vi "address_plus_laserNumber_U32_to_hex.vi"(8 "adress offset":u32=300, 9 "y 3":u32=300) -> (2 "string 5":string)   [LabVIEW 2021]
panel:
  in  "string 6":string
  out "x-y*floor(x/y) 9":u32=2
  out "appended array 3":u32[](array[numeric])
  out "x-y*floor(x/y) 8":u32=2
  out "x-y*floor(x/y) 6":u32=2
  out "x-y*floor(x/y) 7":u32=12
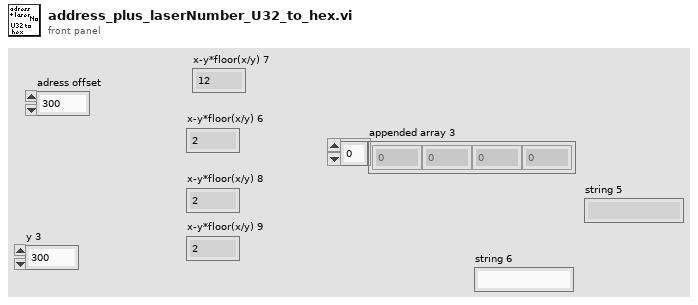
[diagram p1: front panel]
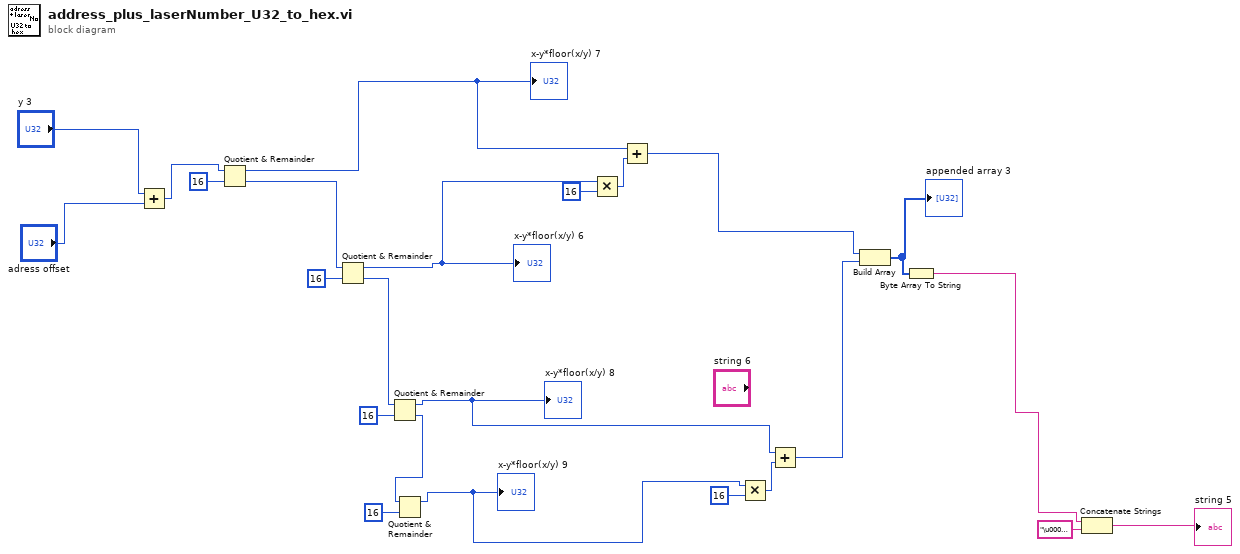
[diagram p0: block diagram]
diagram:
  n1 = Add(x="y 3", y="adress offset") -> (x+y=w6:u32)
  n2 = Quotient & Remainder(x=w6, y=u32 16) -> (x-y*floor(x/y)=w14:u32, floor(x/y)=w24:u32)
  "x-y*floor(x/y) 7" <- w14
  n3 = Quotient & Remainder(x=w24, y=u32 16) -> (x-y*floor(x/y)=w17:u32, floor(x/y)=w20:u32)
  "x-y*floor(x/y) 6" <- w17
  n4 = Quotient & Remainder(x=w20, y=u32 16) -> (x-y*floor(x/y)=w11:u32, floor(x/y)=w18:u32)
  "x-y*floor(x/y) 8" <- w11
  n5 = Quotient & Remainder(x=w18, y=u32 16) -> (x-y*floor(x/y)=w10:u32)  [unwired: 1 out]
  "x-y*floor(x/y) 9" <- w10
  n6 = Multiply(x=w17, y=u32 16) -> (x*y=w15:u32)
  n7 = Add(x=w14, y=w15) -> (x+y=w2:u32)
  n8 = Multiply(x=w10, y=u32 16) -> (x*y=w13:u32)
  n9 = Add(x=w11, y=w13) -> (x+y=w1:u32)
  n10 = Build Array(w2, w1) -> (w9:u32[])
  "appended array 3" <- w9
  n11 = Byte Array To String(unsigned byte array=w9) -> (string=w4:string)
  n12 = Concatenate Strings(w4, "\u0000\u0000" ("string")) -> (→"string 5":string)
